vi "总磷总氮通讯.vi"() -> ()   [LabVIEW 2016, in "斯坦道总氮.lvlib"]
uses:
  <vilib>/Utility/config.llb/NI_LVConfig.lvlib
  <vilib>/Plasmionique/MB Master/MB_Master/MB_Master.lvclass
  <vilib>/Plasmionique/MB Master/MB Master.lvlib
  <vilib>/NI/Modbus Library/API/Wrapper/API Main.lvlib
  <vilib>/NI/Modbus Library/API/Slave/Modbus Slave.lvclass
  <vilib>/NI/Modbus Library/API/Wrapper/Create TCP Slave.vi
  <vilib>/ptbypt/NI_PtbyPt.lvlib
  <vilib>/Utility/config.llb/Write Key (Boolean).vi
  <vilib>/Utility/config.llb/Write Key (String).vi
panel:
  out "氨氮状态告警区":u16[](array[numeric])
  out "氨氮测量数据区":u16[](array[numeric])
  out "COD测量数据区":u16[](array[numeric])
  out "COD状态告警区":u16[](array[numeric])
  out "总氮测量数据区":u16[](array[numeric])
  out "总氮状态告警区":u16[](array[numeric])
  out "总磷状态告警区":u16[](array[numeric])
  out "总磷测量数据区":u16[](array[numeric])
  out "状态告警区":T1 {"告警代码" items=["无告警", "缺试剂告警", "缺水样告警", "缺蒸馏水告警", "缺标液告警", "仪表漏液告警", "标定异常告警", "超量程告警", "加热异常", "低试剂预警", "超上限告警", "超下限告警", "仪表内部其他异常", "滴定异常告警", "电极异常告警", "量程切换告警", "参数设置告警", "PH电极电位异常", "电导率电极异常", "浊度光度异常", "溶解氧电极异常", "溶解氧光强异常", "温度异常告警", "PH异常告警", "溶解氧异常告警", "电导率异常告警", "浊度异常告警", "叶绿素异常告警", "藻密度异常告警", "蓝绿藻异常告警", "ORP异常告警", "氨氮异常告警", "清洁刷异常告警", "SD卡异常告警", "蓝牙异常告警", "Wifi异常告警", "流程异常告警"]; "故障代码" items=["无故障", "电机故障", "温度故障", "通讯故障", "滴定故障"]}
  out "测量数据区":T2 {"单位" items=["ug/L", "mg/L", "ppm", "mg/m3", "cm", "ppb", "ug/m3", "%", "nmol/mol", "umol/mol", "MPN/L", "MPN/100ml", "ng/m3", "NTU", "无量纲", "ms/cm", "us/cm", "℃", "mV", "万个/L"]}
  out "status":bool
  out "关键参数区":T3
  in  "读关键参数区":bool
  in  "读状态告警区":bool
  in  "读测量数据区":bool
  in  "站号":u16(ring) items=["总磷"=1, "氨氮"=3]
  in  "停止":bool
  in  "启动":bool
  in  "控制命令":u16(ring) items=["启动测量"=1, "标样核查"=2, "零点核查"=3, "跨度核查"=4, "空白测试"=5, "平行样测试"=6, "加标回收"=7, "空白校准"=8, "标样校准"=9, "初始化（清洗）"=10, "停止测试"=11, "仪器重启"=12, "校时"=13, "模式设置"=14, "测量间隔设置"=15]
  in  "控制命令参数":u16[](array[numeric]) format="%04xH"
  in  "VISA Resource":refnum<visa-resource-name>
  in  "启用模块":bool
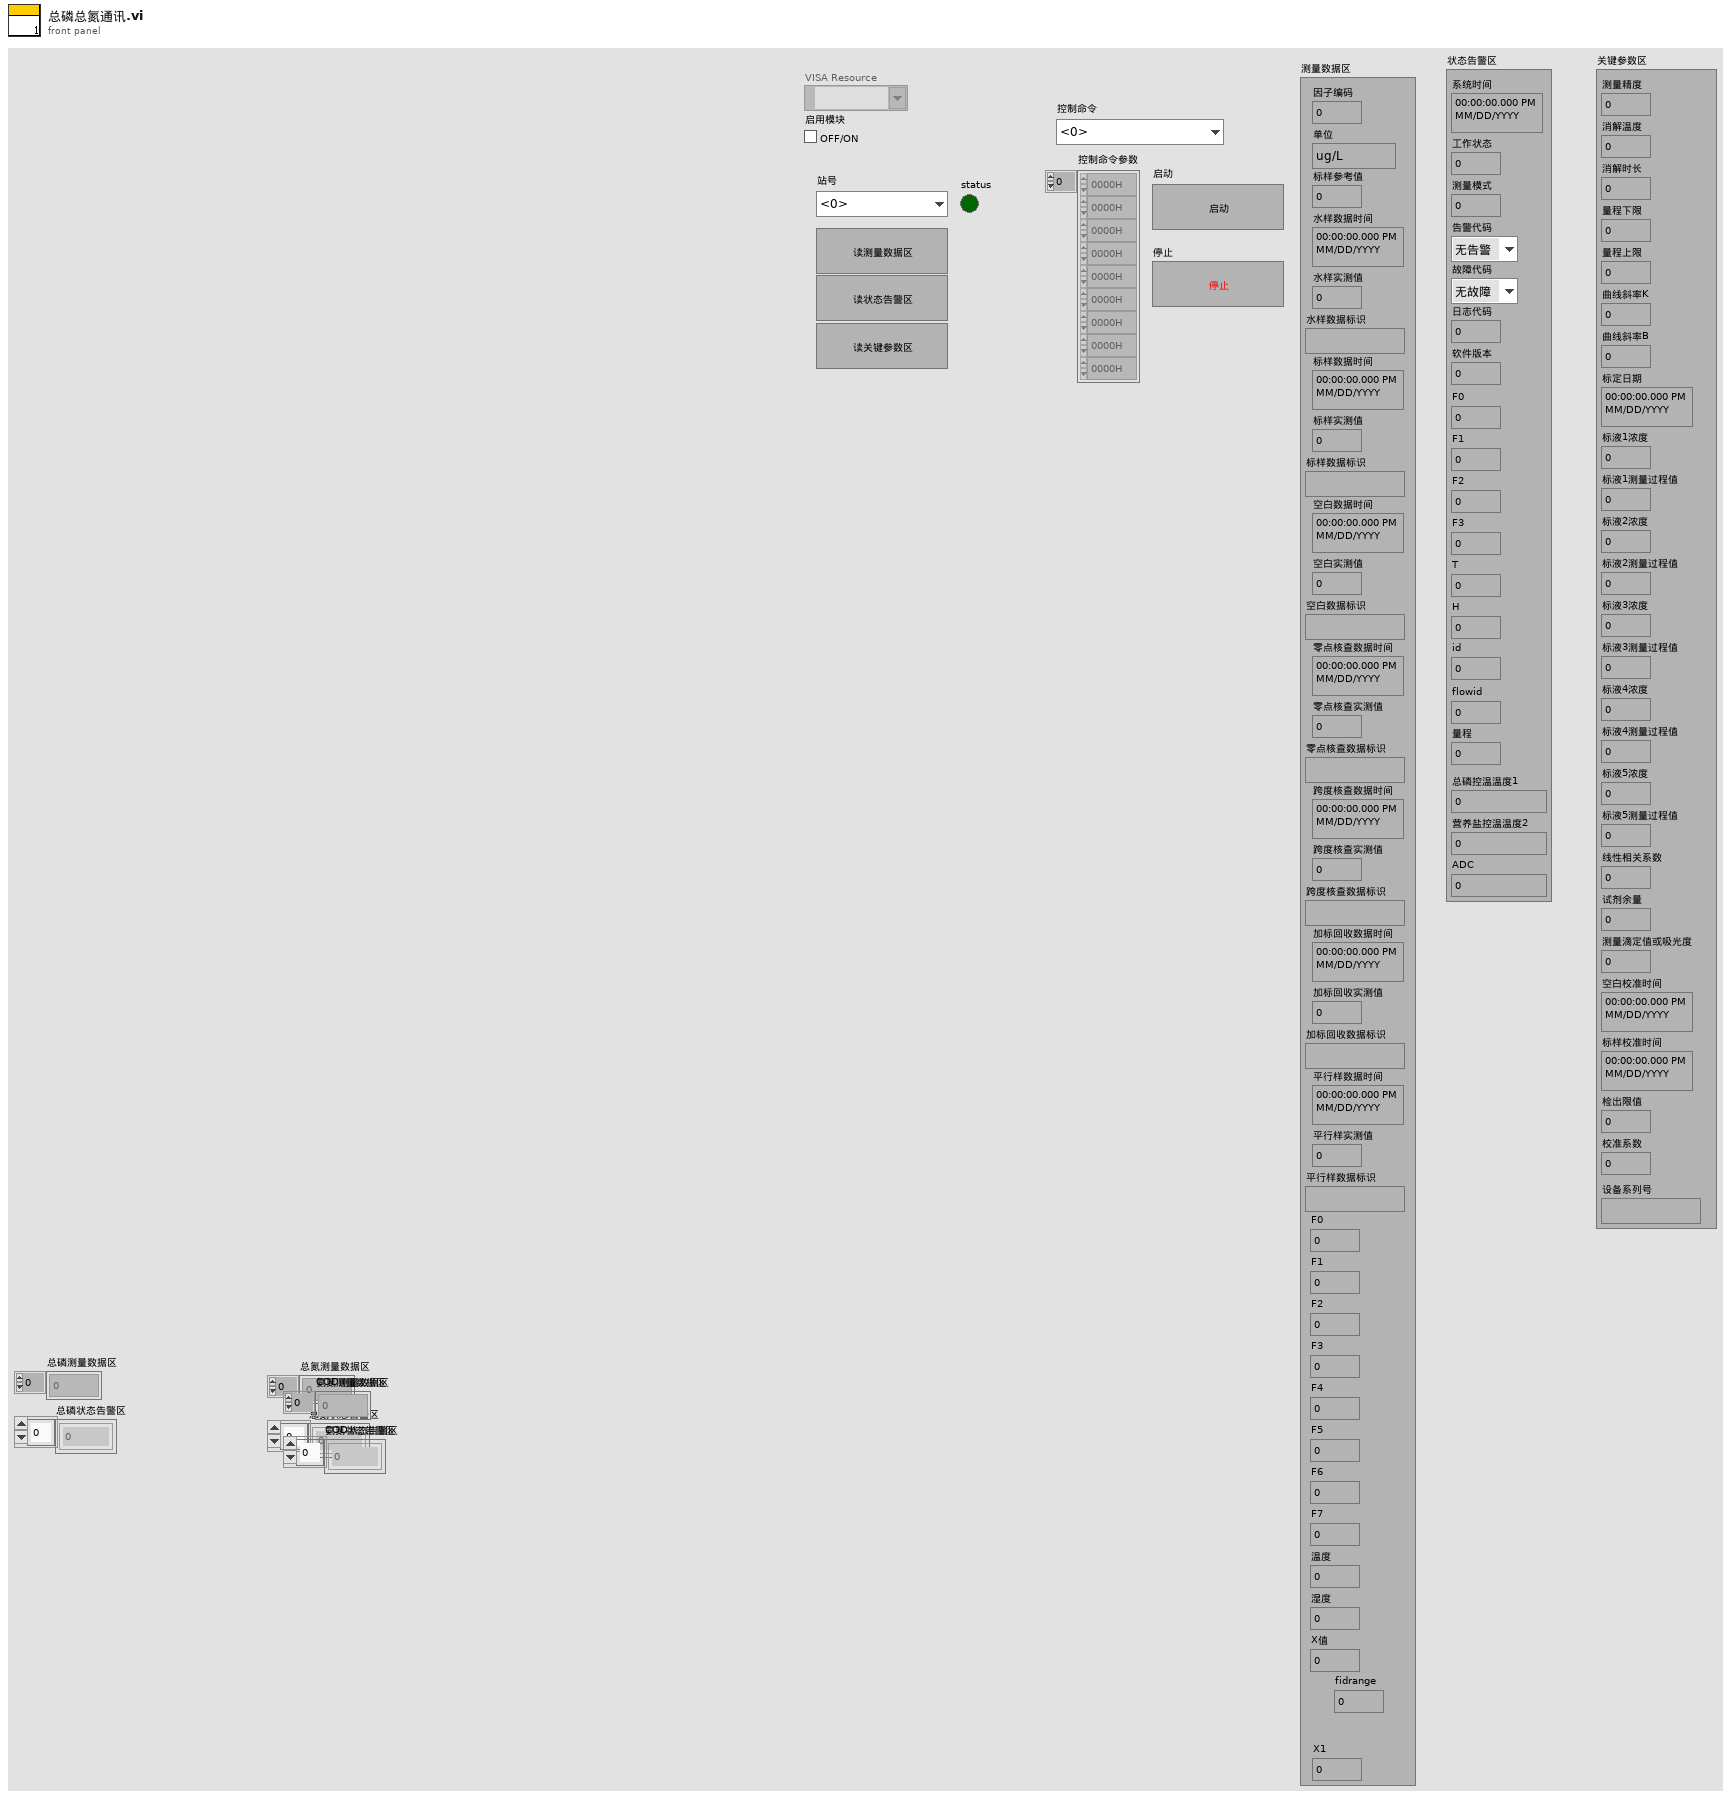
[diagram p1: front panel]
types:
  T1 = cluster{"系统时间":timestamp, "工作状态":u16, "测量模式":u16, "告警代码":u16, "故障代码":u16, "日志代码":u16, "软件版本":u16, "F0":sgl, "F1":sgl, "F2":sgl, "F3":sgl, "T":sgl, "H":sgl, "id":u16, "flowid":u16, "量程":u16, "总磷控温温度1":sgl, "营养盐控温温度2":sgl, "ADC":sgl}
  T2 = cluster{"因子编码":u32, "单位":u16, "标样参考值":sgl, "水样数据时间":timestamp, "水样实测值":sgl, "水样数据标识":string, "标样数据时间":timestamp, "标样实测值":sgl, "标样数据标识":string, "空白数据时间":timestamp, "空白实测值":sgl, "空白数据标识":string, "零点核查数据时间":timestamp, "零点核查实测值":sgl, "零点核查数据标识":string, "跨度核查数据时间":timestamp, "跨度核查实测值":sgl, "跨度核查数据标识":string, "加标回收数据时间":timestamp, "加标回收实测值":sgl, "加标回收数据标识":string, "平行样数据时间":timestamp, "平行样实测值":sgl, "平行样数据标识":string, "F0":sgl, "F1":sgl, "F2":sgl, "F3":sgl, "F4":sgl, "F5":sgl, "F6":sgl, "F7":sgl, "温度":sgl, "湿度":sgl, "X值":sgl, "fidrange":u16, "X1":sgl}
  T3 = cluster{"测量精度":u16, "消解温度":u16, "消解时长":u16, "量程下限":sgl, "量程上限":sgl, "曲线斜率K":sgl, "曲线斜率B":sgl, "标定日期":timestamp, "标液1浓度":sgl, "标液1测量过程值":sgl, "标液2浓度":sgl, "标液2测量过程值":sgl, "标液3浓度":sgl, "标液3测量过程值":sgl, "标液4浓度":sgl, "标液4测量过程值":sgl, "标液5浓度":sgl, "标液5测量过程值":sgl, "线性相关系数":sgl, "试剂余量":u32, "测量滴定值或吸光度":sgl, "空白校准时间":timestamp, "标样校准时间":timestamp, "检出限值":sgl, "校准系数":sgl, "设备系列号":string}
  T4 = cluster{"系统时间":timestamp, "工作状态":u16, "测量模式":enum16{"待机", "连续模式", "周期模式", "定点模式", "受控模式", "手动模式"}, "告警代码":u16, "故障代码":u16, "日志代码":u16, "软件版本":u16, "F0":sgl, "F1":sgl, "F2":sgl, "F3":sgl, "T":sgl, "H":sgl, "id":u16, "flowid":u16, "量程":u16, "总磷控温温度1":sgl, "营养盐控温温度2":sgl, "ADC":sgl}
  T5 = cluster{"因子编码":u32, "单位":u16, "标样参考值":sgl, "水样数据时间":timestamp, "水样实测值":sgl, "水样数据标识":string, "标样数据时间":timestamp, "标样实测值":sgl, "标样数据标识":string, "空白数据时间":timestamp, "空白实测值":sgl, "空白数据标识":string, "零点核查数据时间":timestamp, "零点核查实测值":sgl, "零点核查数据标识":string, "跨度核查数据时间":timestamp, "跨度核查实测值":sgl, "跨度核查数据标识":string, "加标回收数据时间":timestamp, "加标回收实测值":sgl, "加标回收数据标识":string, "平行样数据时间":timestamp, "平行样实测值":sgl, "平行样数据标识":string, "F0":sgl, "F1":sgl, "F2":sgl, "F3":sgl, "F4":sgl, "F5":sgl, "F6":sgl, "F7":sgl, "温度":sgl, "湿度":sgl, "X值":sgl, "fidrange":u16, "X1值":sgl}
  T6 = cluster{"因子编码":u32, "单位":u16, "标样参考值":sgl, "水样数据时间":timestamp, "水样实测值":sgl, "水样数据标识":string, "标样数据时间":timestamp, "标样实测值":sgl, "标样数据标识":string, "空白数据时间":timestamp, "空白实测值":sgl, "空白数据标识":string, "零点核查数据时间":timestamp, "零点核查实测值":sgl, "零点核查数据标识":string, "跨度核查数据时间":timestamp, "跨度核查实测值":sgl, "跨度核查数据标识":string, "加标回收数据时间":timestamp, "加标回收实测值":sgl, "加标回收数据标识":string, "平行样数据时间":timestamp, "平行样实测值":sgl, "平行样数据标识":string, "F0":sgl, "F1":sgl, "F2":sgl, "F3":sgl, "F4":sgl, "F5":sgl, "F6":sgl, "F7":sgl, "温度":sgl, "湿度":sgl, "X值":sgl, "fidrange":u16, "X1值":sgl}[]
  T7 = cluster{"测量精度":u16, "消解温度":u16, "消解时长":u16, "量程下限":sgl, "量程上限":sgl, "曲线斜率K":sgl, "曲线斜率B":sgl, "标定日期":timestamp, "标液1浓度":sgl, "标液1测量过程值":sgl, "标液2浓度":sgl, "标液2测量过程值":sgl, "标液3浓度":sgl, "标液3测量过程值":sgl, "标液4浓度":sgl, "标液4测量过程值":sgl, "标液5浓度":sgl, "标液5测量过程值":sgl, "线性相关系数":sgl, "试剂余量":u32, "测量滴定值或吸光度":sgl, "空白校准时间":timestamp, "标样校准时间":timestamp, "检出限值":sgl, "校准系数":sgl, "设备系列号":string}[]
  T8 = cluster{"系统时间":timestamp, "工作状态":u16, "测量模式":enum16{"待机", "连续模式", "周期模式", "定点模式", "受控模式", "手动模式"}, "告警代码":u16, "故障代码":u16, "日志代码":u16, "软件版本":u16, "F0":sgl, "F1":sgl, "F2":sgl, "F3":sgl, "T":sgl, "H":sgl, "id":u16, "flowid":u16, "量程":u16, "总磷控温温度1":sgl, "营养盐控温温度2":sgl, "ADC":sgl}[]
  T9 = typedef "总磷交互.ctl" = cluster{"状态告警区":cluster{"系统时间":timestamp, "工作状态":u16, "测量模式":enum16{"待机", "连续模式", "周期模式", "定点模式", "受控模式", "手动模式"}, "告警代码":u16, "故障代码":u16, "日志代码":u16, "软件版本":u16, "F0":sgl, "F1":sgl, "F2":sgl, "F3":sgl, "T":sgl, "H":sgl, "id":u16, "flowid":u16, "量程":u16, "总磷控温温度1":sgl, "营养盐控温温度2":sgl, "ADC":sgl}, "平台试剂余量百分比":sgl, "总磷关键参数":T10}
  T10 = typedef "关键参数.ctl" = cluster{"测量量程":sgl, "测量检出限":sgl, "测量精度":sgl, "测量间隔":sgl, "消解温度":sgl, "消解时长":sgl, "三项式系数":sgl, "二次多项式系数":sgl, "曲线斜率":sgl, "曲线截距":sgl, "线性相关系数":sgl, "空白校准时间":timestamp, "标样校准时间":timestamp, "测量信号值":sgl, "稀释倍数":sgl, "空白标定系数":sgl, "量程系数":sgl}
  T11 = typedef "斯坦道总氮.lvlib/关键参数.ctl" = cluster{"测量量程":sgl, "测量检出限":sgl, "测量精度":sgl, "测量间隔":sgl, "消解温度":sgl, "消解时长":sgl, "三项式系数":sgl, "二次多项式系数":sgl, "曲线斜率":sgl, "曲线截距":sgl, "线性相关系数":sgl, "空白校准时间":timestamp, "标样校准时间":timestamp, "测量信号值":sgl, "稀释倍数":sgl, "空白标定系数":sgl, "量程系数":sgl}
  T12 = typedef "总氮交互.ctl" = cluster{"状态告警区":cluster{"系统时间":timestamp, "工作状态":u16, "测量模式":enum16{"待机", "连续模式", "周期模式", "定点模式", "受控模式", "手动模式"}, "告警代码":u16, "故障代码":u16, "日志代码":u16, "软件版本":u16, "F0":sgl, "F1":sgl, "F2":sgl, "F3":sgl, "T":sgl, "H":sgl, "id":u16, "flowid":u16, "量程":u16, "总磷控温温度1":sgl, "营养盐控温温度2":sgl, "ADC":sgl}, "平台试剂余量百分比":sgl, "总氮关键参数":T10}
  T13 = typedef "氨氮交互.ctl" = cluster{"状态告警区":cluster{"系统时间":timestamp, "工作状态":u16, "测量模式":enum16{"待机", "连续模式", "周期模式", "定点模式", "受控模式", "手动模式"}, "告警代码":u16, "故障代码":u16, "日志代码":u16, "软件版本":u16, "F0":sgl, "F1":sgl, "F2":sgl, "F3":sgl, "T":sgl, "H":sgl, "id":u16, "flowid":u16, "量程":u16, "总磷控温温度1":sgl, "营养盐控温温度2":sgl, "ADC":sgl}, "平台试剂余量百分比":sgl, "氨氮关键参数":T10}
  T14 = typedef "CODCr交互.ctl" = cluster{"状态告警区":cluster{"系统时间":timestamp, "工作状态":u16, "测量模式":enum16{"待机", "连续模式", "周期模式", "定点模式", "受控模式", "手动模式"}, "告警代码":u16, "故障代码":u16, "日志代码":u16, "软件版本":u16, "F0":sgl, "F1":sgl, "F2":sgl, "F3":sgl, "T":sgl, "H":sgl, "id":u16, "flowid":u16, "量程":u16, "总磷控温温度1":sgl, "营养盐控温温度2":sgl, "ADC":sgl}, "平台试剂余量百分比":sgl, "CODcr关键参数":T10}
  T15 = typedef "NI_LVConfig.lvlib/Config Data RefNum.ctl" = refnum<k1>
  T16 = enum8{"Enabled", "Disabled", "Disabled and Grayed Out"}
  T17 = cluster{"时间标识":timestamp, "设备":string, "日志信息":string, "备注":string}
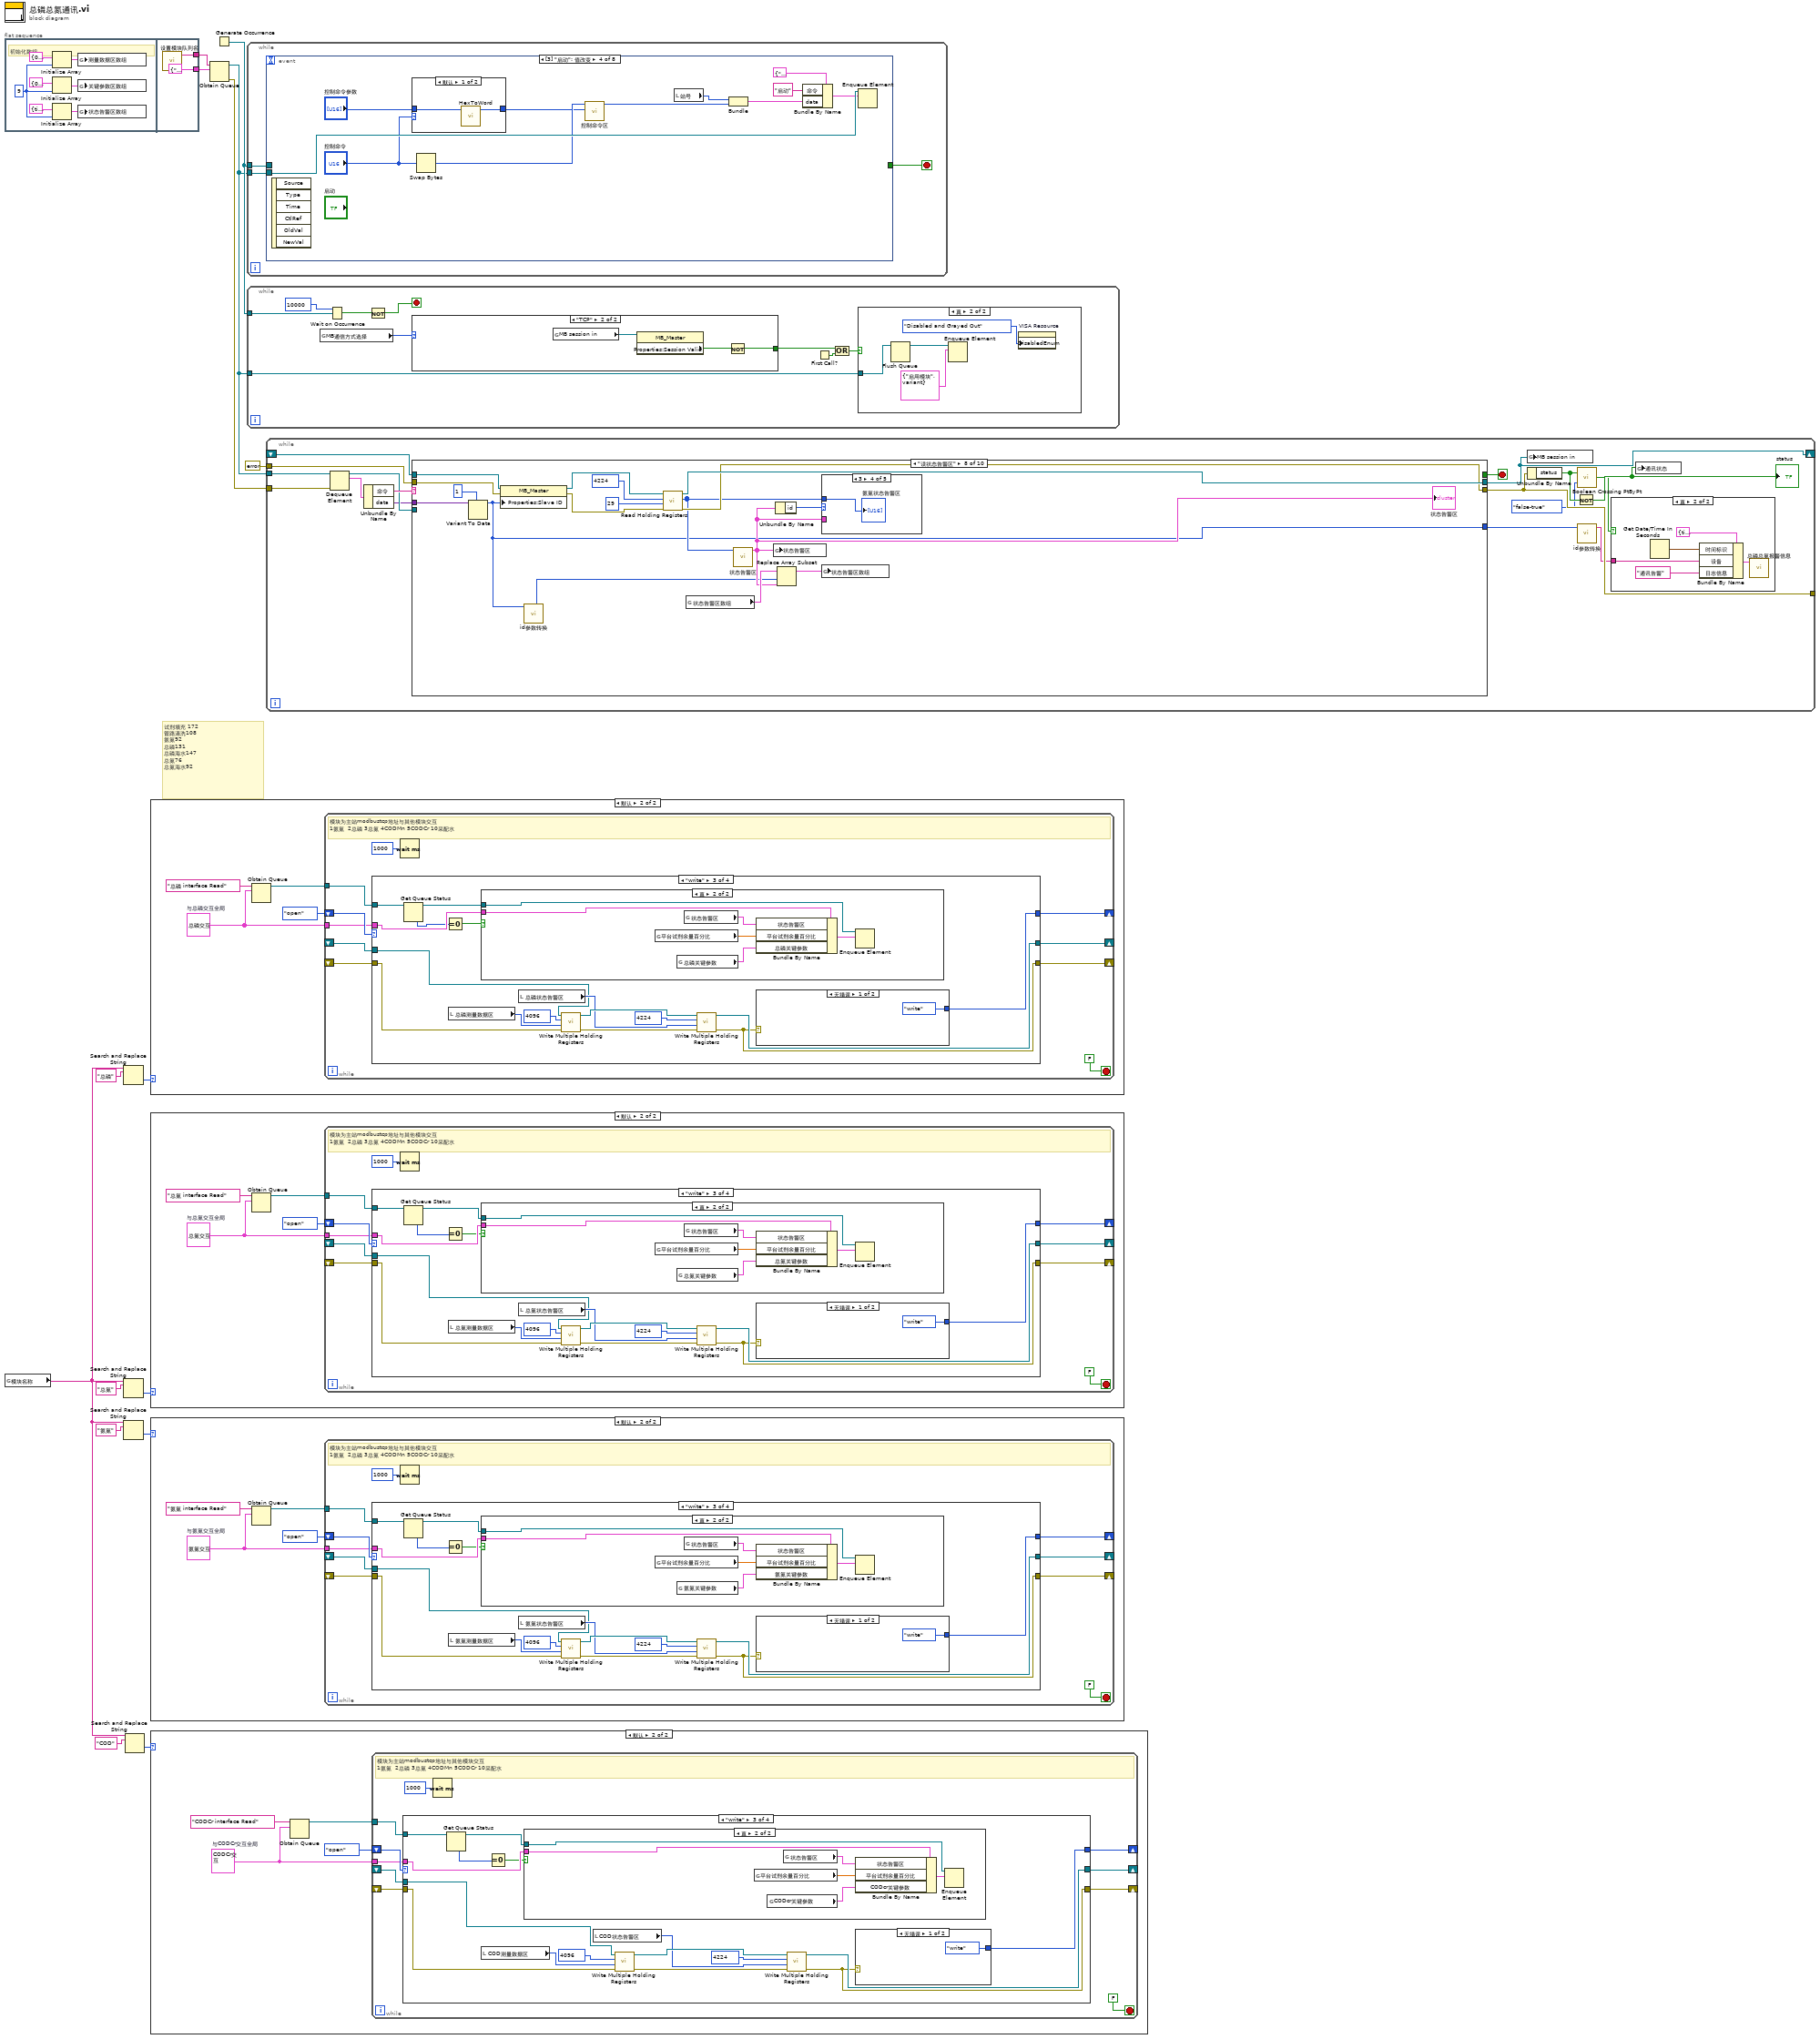
[diagram p0: block diagram]
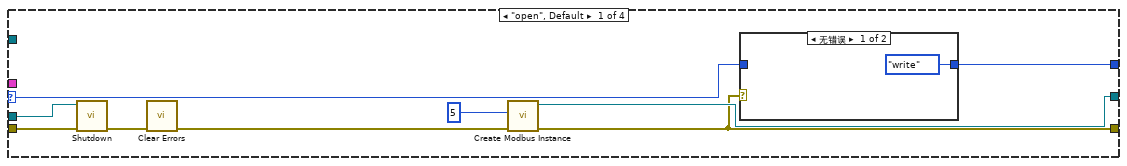
[diagram p3: hidden frame]
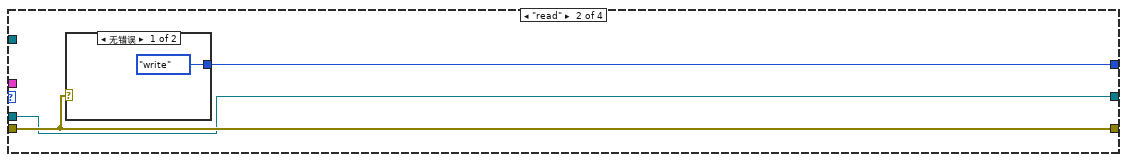
[diagram p5: hidden frame]
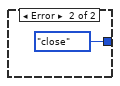
[diagram p6: hidden frame]
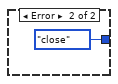
[diagram p8: hidden frame]
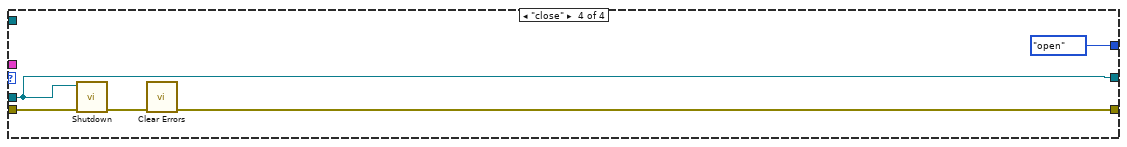
[diagram p9: hidden frame]
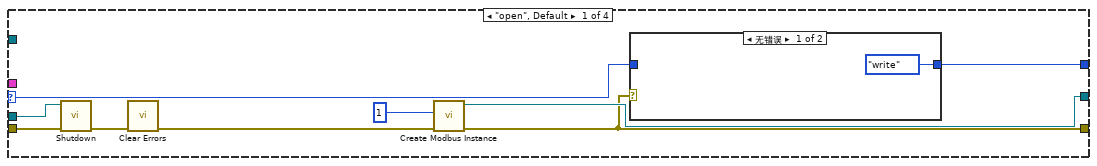
[diagram p11: hidden frame]
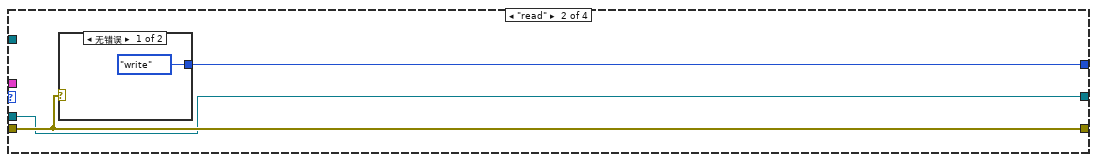
[diagram p13: hidden frame]
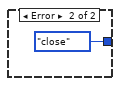
[diagram p14: hidden frame]
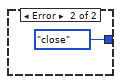
[diagram p16: hidden frame]
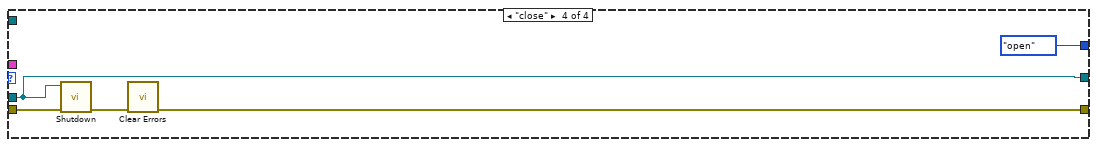
[diagram p17: hidden frame]
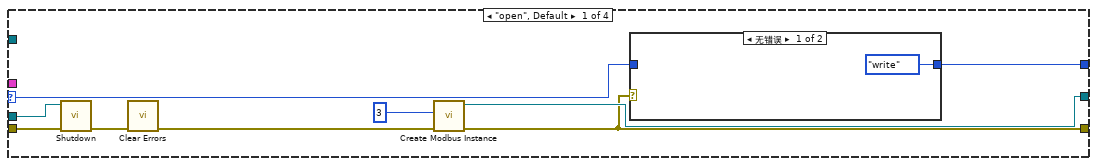
[diagram p19: hidden frame]
diagram:
  # "试剂填充 172 \n管路清洗108\n氨氮92\n总磷131\n总磷海水147\n总氮76\n总氮海水92"
  n1 = flat-sequence {
    tunnel: [cluster{"命令":string, "data":variant} {"命令"="", "data"=variant}] -> w15
    tunnel: [w23] -> w10
    frame #0 {
      w16 = 9 ("维数大小")
      # "初始化数组"
      n2 = Initialize Array(T5 {"因子编码"=0, "单位"=0, "标样参考值"=0.0, "水样数据时间"=timestamp(0 s since 1904-01-01), "水样实测值"=0.0, "水样数据标识"="", "标样数据时间"=timestamp(0 s since 1904-01-01), "标样实测值"=0.0, "标样数据标识"="", "空白数据时间"=timestamp(0 s since 1904-01-01), "空白实测值"=0.0, "空白数据标识"="", "零点核查数据时间"=timestamp(0 s since 1904-01-01), "零点核查实测值"=0.0, "零点核查数据标识"="", "跨度核查数据时间"=timestamp(0 s since 1904-01-01), "跨度核查实测值"=0.0, "跨度核查数据标识"="", "加标回收数据时间"=timestamp(0 s since 1904-01-01), "加标回收实测值"=0.0, "加标回收数据标识"="", "平行样数据时间"=timestamp(0 s since 1904-01-01), "平行样实测值"=0.0, "平行样数据标识"="", "F0"=0.0, "F1"=0.0, "F2"=0.0, "F3"=0.0, "F4"=0.0, "F5"=0.0, "F6"=0.0, "F7"=0.0, "温度"=0.0, "湿度"=0.0, "X值"=0.0, "fidrange"=0, "X1值"=0.0} ("测量数据区"), w16) -> (w22:T6)
      n3 = Initialize Array(T3 {"测量精度"=0, "消解温度"=0, "消解时长"=0, "量程下限"=0.0, "量程上限"=0.0, "曲线斜率K"=0.0, "曲线斜率B"=0.0, "标定日期"=timestamp(0 s since 1904-01-01), "标液1浓度"=0.0, "标液1测量过程值"=0.0, "标液2浓度"=0.0, "标液2测量过程值"=0.0, "标液3浓度"=0.0, "标液3测量过程值"=0.0, "标液4浓度"=0.0, "标液4测量过程值"=0.0, "标液5浓度"=0.0, "标液5测量过程值"=0.0, "线性相关系数"=0.0, "试剂余量"=0, "测量滴定值或吸光度"=0.0, "空白校准时间"=timestamp(0 s since 1904-01-01), "标样校准时间"=timestamp(0 s since 1904-01-01), "检出限值"=0.0, "校准系数"=0.0, "设备系列号"=""} ("关键参数区"), w16) -> (w20:T7)
      n4 = Initialize Array(T4 {"系统时间"=timestamp(0 s since 1904-01-01), "工作状态"=0, "测量模式"=enum."待机", "告警代码"=0, "故障代码"=0, "日志代码"=0, "软件版本"=0, "F0"=0.0, "F1"=0.0, "F2"=0.0, "F3"=0.0, "T"=0.0, "H"=0.0, "id"=0, "flowid"=0, "量程"=0, "总磷控温温度1"=0.0, "营养盐控温温度2"=0.0, "ADC"=0.0} ("状态告警区"), w16) -> (w19:T8)
      n5 = global write "VAR总磷总氮全局变量.vi" "测量数据区数组"(w22) -> ()
      n6 = global write "VAR总磷总氮全局变量.vi" "关键参数区数组"(w20) -> ()
      n7 = global write "VAR总磷总氮全局变量.vi" "状态告警区数组"(w19) -> ()
    }
    frame #1 {
      n8 = call "设置模块队列名.vi"() -> ("Msg"=w23:string)  [unwired: 5 in]
    }
  }
  n9 = global read "VAR总磷总氮全局变量.vi" "模块名称"() -> (w3:string)
  n10 = Search and Replace String(input string=w3, search string="总磷" ("搜索字符串")) -> (offset past replacement=w8:i32)  [unwired: 6 in, 3 out]
  n11 = Search and Replace String(input string=w3, search string="总氮" ("搜索字符串")) -> (offset past replacement=w6:i32)  [unwired: 6 in, 3 out]
  n12 = Search and Replace String(input string=w3, search string="氨氮" ("搜索字符串")) -> (offset past replacement=w4:i32)  [unwired: 6 in, 3 out]
  n13 = Search and Replace String(input string=w3, search string="COD" ("搜索字符串")) -> (offset past replacement=w1:i32)  [unwired: 6 in, 3 out]
  n14 = case shown="默认" w8 {
    frame -1 {
    }
    frame Default {
      w25 = T9 {"状态告警区"={"系统时间"=timestamp(0 s since 1904-01-01), "工作状态"=0, "测量模式"=enum."待机", "告警代码"=0, "故障代码"=0, "日志代码"=0, "软件版本"=0, "F0"=0.0, "F1"=0.0, "F2"=0.0, "F3"=0.0, "T"=0.0, "H"=0.0, "id"=0, "flowid"=0, "量程"=0, "总磷控温温度1"=0.0, "营养盐控温温度2"=0.0, "ADC"=0.0}, "平台试剂余量百分比"=0.0, "总磷关键参数"={"测量量程"=0.0, "测量检出限"=0.0, "测量精度"=0.0, "测量间隔"=0.0, "消解温度"=0.0, "消解时长"=0.0, "三项式系数"=0.0, "二次多项式系数"=0.0, "曲线斜率"=0.0, "曲线截距"=0.0, "线性相关系数"=0.0, "空白校准时间"=timestamp(0 s since 1904-01-01), "标样校准时间"=timestamp(0 s since 1904-01-01), "测量信号值"=0.0, "稀释倍数"=0.0, "空白标定系数"=0.0, "量程系数"=0.0}}  # 与总磷交互全局
      n15 = Obtain Queue(name (unnamed)="总磷 interface Read" ("写入方名称"), element data type=w25) -> (queue out=w26:refnum<queue>)  [unwired: 3 in, 2 out]
      n16 = while {
        shift-right: [w36] -> _
        shift-left: _ -> [w38]
        shift-right: [w35] -> _
        shift-left: _ -> [w37]
        shift-right: [w32] -> _
        shift-left: enum16{"open", "read", "write", "close"}."open" -> [w33]
        tunnel: w26 -> [w30]
        tunnel: w25 -> [w29]
        stop <- FALSE stop-if-true
        # "模块为主站modbustcp地址与其他模块交互\n1氨氮  2总磷 3总氮 4CODMn 5CODCr 10采配水"
        n17 = case shown="\"write\"" w33 {
          selector: w33 -> [w47 _ _ _]
          tunnel: w38 -> [w41 w50 w61 w81]
          tunnel: w37 -> [w40 w51 w60 w80]
          tunnel: [w44 w50 w66 w81] -> w36
          tunnel: [w43 w51 w65 w83] -> w35
          tunnel: [w46 w52 w70 enum16{"open", "read", "write", "close"}."open"] -> w32
          tunnel: w30 -> [_ _ w59 _]
          tunnel: w29 -> [_ _ w58 _]
          frame "open", Default {
            n18 = call-dynamic "Shutdown.vi"("error in"=w40, "Modbus slave in"=w41) -> ("error out"=w39:errorcluster)  [unwired: 9 in]
            n19 = call <vilib>:"Clear Errors.vi"("error in (no error)"=w39) -> ("error out"=w42:errorcluster)  [unwired: 5 in, 1 out]
            n20 = call-poly <vilib>:"Create Modbus Instance.vi"("error in"=w42, "port (502)"=u16 2) -> ("error out"=w43:errorcluster, "TCP slave instance"=w44:refnum<class "Modbus Slave.lvclass">)  [unwired: 8 in]
            n21 = case shown="无错误" w43 {
              tunnel: w47 -> [_ w49]
              tunnel: [enum16{"open", "read", "write", "close"}."write" w49] -> w46
              frame No Error {
              }
              frame Error {
              }
            }
          }
          frame "read" {
            n22 = case shown="无错误" w51 {
              tunnel: [enum16{"open", "read", "write", "close"}."write" enum16{"open", "read", "write", "close"}."close"] -> w52
              frame No Error {
              }
              frame Error {
              }
            }
          }
          frame "write" {
            n23 = Get Queue Status(queue=w59) -> (queue out=w57:refnum<queue>, # elements in queue=w56:i32)  [unwired: 2 in, 6 out]
            n24 = Equal To 0?(x=w56) -> (x = 0?=w55:bool)
            n25 = local read "总磷测量数据区"() -> (w64:u16[])
            n26 = case shown="真" w55 {
              tunnel: w58 -> [_ w73]
              tunnel: w57 -> [_ w71]
              frame False {
              }
              frame True {
                n27 = global read "VAR总磷总氮全局变量.vi" "平台试剂余量百分比"() -> (w75:sgl)
                n28 = global read "VAR总磷总氮全局变量.vi" "总磷关键参数"() -> (w76:T11)
                n29 = global read "VAR总磷总氮全局变量.vi" "状态告警区"() -> (w74:T4)
                n30 = Bundle By Name(cluster=w73, "状态告警区"=w74, "平台试剂余量百分比"=w75, "总磷关键参数"=w76) -> (w72:T9)
                n31 = Enqueue Element(queue=w71, element=w72) -> ()  [unwired: 2 in, 3 out]
              }
            }
            n32 = local read "总磷状态告警区"() -> (w62:u16[])
            n33 = call-dynamic "Write Multiple Holding Registers.vi"("error in"=w60, "registers to write"=w64, "starting address"=u16 4096, "Modbus slave in"=w61) -> ("error out"=w67:errorcluster, "Modbus slave out"=w68:refnum<class "Modbus Slave.lvclass">)  [unwired: 6 in]
            n34 = call-dynamic "Write Multiple Holding Registers.vi"("error in"=w67, "registers to write"=w62, "starting address"=u16 4224, "Modbus slave in"=w68) -> ("error out"=w65:errorcluster, "Modbus slave out"=w66:refnum<class "Modbus Slave.lvclass">)  [unwired: 6 in]
            n35 = case shown="无错误" w65 {
              tunnel: [enum16{"open", "read", "write", "close"}."write" enum16{"open", "read", "write", "close"}."close"] -> w70
              frame No Error {
              }
              frame Error {
              }
            }
          }
          frame "close" {
            n36 = call-dynamic "Shutdown.vi"("error in"=w80, "Modbus slave in"=w81) -> ("error out"=w79:errorcluster)  [unwired: 9 in]
            n37 = call <vilib>:"Clear Errors.vi"("error in (no error)"=w79) -> ("error out"=w83:errorcluster)  [unwired: 5 in, 1 out]
          }
        }
        n38 = Wait (ms)(milliseconds to wait=u32 1000 ("等待时间（毫秒）")) -> ()  [unwired: 1 out]
      }
    }
  }
  n39 = case shown="默认" w6 {
    frame -1 {
    }
    frame Default {
      w84 = T12 {"状态告警区"={"系统时间"=timestamp(0 s since 1904-01-01), "工作状态"=0, "测量模式"=enum."待机", "告警代码"=0, "故障代码"=0, "日志代码"=0, "软件版本"=0, "F0"=0.0, "F1"=0.0, "F2"=0.0, "F3"=0.0, "T"=0.0, "H"=0.0, "id"=0, "flowid"=0, "量程"=0, "总磷控温温度1"=0.0, "营养盐控温温度2"=0.0, "ADC"=0.0}, "平台试剂余量百分比"=0.0, "总氮关键参数"={"测量量程"=0.0, "测量检出限"=0.0, "测量精度"=0.0, "测量间隔"=0.0, "消解温度"=0.0, "消解时长"=0.0, "三项式系数"=0.0, "二次多项式系数"=0.0, "曲线斜率"=0.0, "曲线截距"=0.0, "线性相关系数"=0.0, "空白校准时间"=timestamp(0 s since 1904-01-01), "标样校准时间"=timestamp(0 s since 1904-01-01), "测量信号值"=0.0, "稀释倍数"=0.0, "空白标定系数"=0.0, "量程系数"=0.0}}  # 与总氮交互全局
      n40 = Obtain Queue(name (unnamed)="总氮 interface Read" ("写入方名称"), element data type=w84) -> (queue out=w85:refnum<queue>)  [unwired: 3 in, 2 out]
      n41 = while {
        shift-right: [w95] -> _
        shift-left: _ -> [w97]
        shift-right: [w94] -> _
        shift-left: _ -> [w96]
        shift-right: [w91] -> _
        shift-left: enum16{"open", "read", "write", "close"}."open" -> [w92]
        tunnel: w85 -> [w89]
        tunnel: w84 -> [w88]
        stop <- FALSE stop-if-true
        # "模块为主站modbustcp地址与其他模块交互\n1氨氮  2总磷 3总氮 4CODMn 5CODCr 10采配水"
        n42 = case shown="\"write\"" w92 {
          selector: w92 -> [w106 _ _ _]
          tunnel: w97 -> [w100 w109 w120 w140]
          tunnel: w96 -> [w99 w110 w119 w139]
          tunnel: [w103 w109 w125 w140] -> w95
          tunnel: [w102 w110 w124 w142] -> w94
          tunnel: [w105 w111 w129 enum16{"open", "read", "write", "close"}."open"] -> w91
          tunnel: w89 -> [_ _ w118 _]
          tunnel: w88 -> [_ _ w117 _]
          frame "open", Default {
            n43 = call-dynamic "Shutdown.vi"("error in"=w99, "Modbus slave in"=w100) -> ("error out"=w98:errorcluster)  [unwired: 9 in]
            n44 = call <vilib>:"Clear Errors.vi"("error in (no error)"=w98) -> ("error out"=w101:errorcluster)  [unwired: 5 in, 1 out]
            n45 = call-poly <vilib>:"Create Modbus Instance.vi"("error in"=w101, "port (502)"=u16 3) -> ("error out"=w102:errorcluster, "TCP slave instance"=w103:refnum<class "Modbus Slave.lvclass">)  [unwired: 8 in]
            n46 = case shown="无错误" w102 {
              tunnel: w106 -> [_ w108]
              tunnel: [enum16{"open", "read", "write", "close"}."write" w108] -> w105
              frame No Error {
              }
              frame Error {
              }
            }
          }
          frame "read" {
            n47 = case shown="无错误" w110 {
              tunnel: [enum16{"open", "read", "write", "close"}."write" enum16{"open", "read", "write", "close"}."close"] -> w111
              frame No Error {
              }
              frame Error {
              }
            }
          }
          frame "write" {
            n48 = Get Queue Status(queue=w118) -> (queue out=w116:refnum<queue>, # elements in queue=w115:i32)  [unwired: 2 in, 6 out]
            n49 = Equal To 0?(x=w115) -> (x = 0?=w114:bool)
            n50 = local read "总氮测量数据区"() -> (w123:u16[])
            n51 = case shown="真" w114 {
              tunnel: w116 -> [_ w131]
              tunnel: w117 -> [_ w130]
              frame False {
              }
              frame True {
                n52 = global read "VAR总磷总氮全局变量.vi" "平台试剂余量百分比"() -> (w134:sgl)
                n53 = global read "VAR总磷总氮全局变量.vi" "总氮关键参数"() -> (w135:T11)
                n54 = global read "VAR总磷总氮全局变量.vi" "状态告警区"() -> (w133:T4)
                n55 = Bundle By Name(cluster=w130, "状态告警区"=w133, "平台试剂余量百分比"=w134, "总氮关键参数"=w135) -> (w132:T12)
                n56 = Enqueue Element(queue=w131, element=w132) -> ()  [unwired: 2 in, 3 out]
              }
            }
            n57 = local read "总氮状态告警区"() -> (w121:u16[])
            n58 = call-dynamic "Write Multiple Holding Registers.vi"("error in"=w119, "registers to write"=w123, "starting address"=u16 4096, "Modbus slave in"=w120) -> ("error out"=w126:errorcluster, "Modbus slave out"=w127:refnum<class "Modbus Slave.lvclass">)  [unwired: 6 in]
            n59 = call-dynamic "Write Multiple Holding Registers.vi"("error in"=w126, "registers to write"=w121, "starting address"=u16 4224, "Modbus slave in"=w127) -> ("error out"=w124:errorcluster, "Modbus slave out"=w125:refnum<class "Modbus Slave.lvclass">)  [unwired: 6 in]
            n60 = case shown="无错误" w124 {
              tunnel: [enum16{"open", "read", "write", "close"}."write" enum16{"open", "read", "write", "close"}."close"] -> w129
              frame No Error {
              }
              frame Error {
              }
            }
          }
          frame "close" {
            n61 = call-dynamic "Shutdown.vi"("error in"=w139, "Modbus slave in"=w140) -> ("error out"=w138:errorcluster)  [unwired: 9 in]
            n62 = call <vilib>:"Clear Errors.vi"("error in (no error)"=w138) -> ("error out"=w142:errorcluster)  [unwired: 5 in, 1 out]
          }
        }
        n63 = Wait (ms)(milliseconds to wait=u32 1000 ("等待时间（毫秒）")) -> ()  [unwired: 1 out]
      }
    }
  }
  n64 = case shown="默认" w4 {
    frame -1 {
    }
    frame Default {
      w143 = T13 {"状态告警区"={"系统时间"=timestamp(0 s since 1904-01-01), "工作状态"=0, "测量模式"=enum."待机", "告警代码"=0, "故障代码"=0, "日志代码"=0, "软件版本"=0, "F0"=0.0, "F1"=0.0, "F2"=0.0, "F3"=0.0, "T"=0.0, "H"=0.0, "id"=0, "flowid"=0, "量程"=0, "总磷控温温度1"=0.0, "营养盐控温温度2"=0.0, "ADC"=0.0}, "平台试剂余量百分比"=0.0, "氨氮关键参数"={"测量量程"=0.0, "测量检出限"=0.0, "测量精度"=0.0, "测量间隔"=0.0, "消解温度"=0.0, "消解时长"=0.0, "三项式系数"=0.0, "二次多项式系数"=0.0, "曲线斜率"=0.0, "曲线截距"=0.0, "线性相关系数"=0.0, "空白校准时间"=timestamp(0 s since 1904-01-01), "标样校准时间"=timestamp(0 s since 1904-01-01), "测量信号值"=0.0, "稀释倍数"=0.0, "空白标定系数"=0.0, "量程系数"=0.0}}  # 与氨氮交互全局
      n65 = Obtain Queue(name (unnamed)="氨氮 interface Read" ("写入方名称"), element data type=w143) -> (queue out=w144:refnum<queue>)  [unwired: 3 in, 2 out]
      n66 = while {
        shift-right: [w154] -> _
        shift-left: _ -> [w156]
        shift-right: [w153] -> _
        shift-left: _ -> [w155]
        shift-right: [w150] -> _
        shift-left: enum16{"open", "read", "write", "close"}."open" -> [w151]
        tunnel: w144 -> [w148]
        tunnel: w143 -> [w147]
        stop <- FALSE stop-if-true
        # "模块为主站modbustcp地址与其他模块交互\n1氨氮  2总磷 3总氮 4CODMn 5CODCr 10采配水"
        n67 = case shown="\"write\"" w151 {
          selector: w151 -> [w165 _ _ _]
          tunnel: w156 -> [w159 w168 w179 w199]
          tunnel: w155 -> [w158 w169 w178 w198]
          tunnel: [w162 w168 w184 w199] -> w154
          tunnel: [w161 w169 w183 w201] -> w153
          tunnel: [w164 w170 w188 enum16{"open", "read", "write", "close"}."open"] -> w150
          tunnel: w148 -> [_ _ w175 _]
          tunnel: w147 -> [_ _ w177 _]
          frame "open", Default {
            n68 = call-dynamic "Shutdown.vi"("error in"=w158, "Modbus slave in"=w159) -> ("error out"=w157:errorcluster)  [unwired: 9 in]
            n69 = call <vilib>:"Clear Errors.vi"("error in (no error)"=w157) -> ("error out"=w160:errorcluster)  [unwired: 5 in, 1 out]
            n70 = call-poly <vilib>:"Create Modbus Instance.vi"("error in"=w160, "port (502)"=u16 1) -> ("error out"=w161:errorcluster, "TCP slave instance"=w162:refnum<class "Modbus Slave.lvclass">)  [unwired: 8 in]
            n71 = case shown="无错误" w161 {
              tunnel: w165 -> [_ w167]
              tunnel: [enum16{"open", "read", "write", "close"}."write" w167] -> w164
              frame No Error {
              }
              frame Error {
              }
            }
          }
          frame "read" {
            n72 = case shown="无错误" w169 {
              tunnel: [enum16{"open", "read", "write", "close"}."write" enum16{"open", "read", "write", "close"}."close"] -> w170
              frame No Error {
              }
              frame Error {
              }
            }
          }
          frame "write" {
            n73 = Get Queue Status(queue=w175) -> (queue out=w174:refnum<queue>, # elements in queue=w176:i32)  [unwired: 2 in, 6 out]
            n74 = Equal To 0?(x=w176) -> (x = 0?=w173:bool)
            n75 = local read "氨氮测量数据区"() -> (w182:u16[])
            n76 = case shown="真" w173 {
              tunnel: w174 -> [_ w190]
              tunnel: w177 -> [_ w189]
              frame False {
              }
              frame True {
                n77 = global read "VAR总磷总氮全局变量.vi" "平台试剂余量百分比"() -> (w193:sgl)
                n78 = global read "VAR总磷总氮全局变量.vi" "氨氮关键参数"() -> (w194:T11)
                n79 = global read "VAR总磷总氮全局变量.vi" "状态告警区"() -> (w192:T4)
                n80 = Bundle By Name(cluster=w189, "状态告警区"=w192, "平台试剂余量百分比"=w193, "氨氮关键参数"=w194) -> (w191:T13)
                n81 = Enqueue Element(queue=w190, element=w191) -> ()  [unwired: 2 in, 3 out]
              }
            }
            n82 = local read "氨氮状态告警区"() -> (w180:u16[])
            n83 = call-dynamic "Write Multiple Holding Registers.vi"("error in"=w178, "registers to write"=w182, "starting address"=u16 4096, "Modbus slave in"=w179) -> ("error out"=w185:errorcluster, "Modbus slave out"=w186:refnum<class "Modbus Slave.lvclass">)  [unwired: 6 in]
            n84 = call-dynamic "Write Multiple Holding Registers.vi"("error in"=w185, "registers to write"=w180, "starting address"=u16 4224, "Modbus slave in"=w186) -> ("error out"=w183:errorcluster, "Modbus slave out"=w184:refnum<class "Modbus Slave.lvclass">)  [unwired: 6 in]
            n85 = case shown="无错误" w183 {
              tunnel: [enum16{"open", "read", "write", "close"}."write" enum16{"open", "read", "write", "close"}."close"] -> w188
              frame No Error {
              }
              frame Error {
              }
            }
          }
          frame "close" {
            n86 = call-dynamic "Shutdown.vi"("error in"=w198, "Modbus slave in"=w199) -> ("error out"=w197:errorcluster)  [unwired: 9 in]
            n87 = call <vilib>:"Clear Errors.vi"("error in (no error)"=w197) -> ("error out"=w201:errorcluster)  [unwired: 5 in, 1 out]
          }
        }
        n88 = Wait (ms)(milliseconds to wait=u32 1000 ("等待时间（毫秒）")) -> ()  [unwired: 1 out]
      }
    }
  }
  n89 = case shown="默认" w1 {
    frame -1 {
    }
    frame Default {
      w203 = T14 {"状态告警区"={"系统时间"=timestamp(0 s since 1904-01-01), "工作状态"=0, "测量模式"=enum."待机", "告警代码"=0, "故障代码"=0, "日志代码"=0, "软件版本"=0, "F0"=0.0, "F1"=0.0, "F2"=0.0, "F3"=0.0, "T"=0.0, "H"=0.0, "id"=0, "flowid"=0, "量程"=0, "总磷控温温度1"=0.0, "营养盐控温温度2"=0.0, "ADC"=0.0}, "平台试剂余量百分比"=0.0, "CODcr关键参数"={"测量量程"=0.0, "测量检出限"=0.0, "测量精度"=0.0, "测量间隔"=0.0, "消解温度"=0.0, "消解时长"=0.0, "三项式系数"=0.0, "二次多项式系数"=0.0, "曲线斜率"=0.0, "曲线截距"=0.0, "线性相关系数"=0.0, "空白校准时间"=timestamp(0 s since 1904-01-01), "标样校准时间"=timestamp(0 s since 1904-01-01), "测量信号值"=0.0, "稀释倍数"=0.0, "空白标定系数"=0.0, "量程系数"=0.0}}  # 与CODCr交互全局
      n90 = Obtain Queue(name (unnamed)="CODCr interface Read" ("写入方名称"), element data type=w203) -> (queue out=w204:refnum<queue>)  [unwired: 3 in, 2 out]
      n91 = while {
        shift-right: [w213] -> _
        shift-left: _ -> [w215]
        shift-right: [w212] -> _
        shift-left: _ -> [w214]
        shift-right: [w209] -> _
        shift-left: enum16{"open", "read", "write", "close"}."open" -> [w210]
        tunnel: w204 -> [w207]
        tunnel: w203 -> [w206]
        stop <- FALSE stop-if-true
        # "模块为主站modbustcp地址与其他模块交互\n1氨氮  2总磷 3总氮 4CODMn 5CODCr 10采配水"
        n92 = case shown="\"write\"" w210 {
          selector: w210 -> [w224 _ _ _]
          tunnel: w215 -> [w218 w227 w238 w258]
          tunnel: w214 -> [w217 w228 w237 w257]
          tunnel: [w221 w227 w243 w258] -> w213
          tunnel: [w220 w228 w242 w260] -> w212
          tunnel: [w223 w229 w247 enum16{"open", "read", "write", "close"}."open"] -> w209
          tunnel: w207 -> [_ _ w234 _]
          tunnel: w206 -> [_ _ w236 _]
          frame "open", Default {
            n93 = call-dynamic "Shutdown.vi"("error in"=w217, "Modbus slave in"=w218) -> ("error out"=w216:errorcluster)  [unwired: 9 in]
            n94 = call <vilib>:"Clear Errors.vi"("error in (no error)"=w216) -> ("error out"=w219:errorcluster)  [unwired: 5 in, 1 out]
            n95 = call-poly <vilib>:"Create Modbus Instance.vi"("error in"=w219, "port (502)"=u16 5) -> ("error out"=w220:errorcluster, "TCP slave instance"=w221:refnum<class "Modbus Slave.lvclass">)  [unwired: 8 in]
            n96 = case shown="无错误" w220 {
              tunnel: w224 -> [_ w226]
              tunnel: [enum16{"open", "read", "write", "close"}."write" w226] -> w223
              frame No Error {
              }
              frame Error {
              }
            }
          }
          frame "read" {
            n97 = case shown="无错误" w228 {
              tunnel: [enum16{"open", "read", "write", "close"}."write" enum16{"open", "read", "write", "close"}."close"] -> w229
              frame No Error {
              }
              frame Error {
              }
            }
          }
          frame "write" {
            n98 = Get Queue Status(queue=w234) -> (queue out=w233:refnum<queue>, # elements in queue=w235:i32)  [unwired: 2 in, 6 out]
            n99 = local read "COD测量数据区"() -> (w241:u16[])
            n100 = Equal To 0?(x=w235) -> (x = 0?=w232:bool)
            n101 = case shown="真" w232 {
              tunnel: w233 -> [_ w249]
              tunnel: w236 -> [_ w248]
              frame False {
              }
              frame True {
                n102 = global read "VAR总磷总氮全局变量.vi" "平台试剂余量百分比"() -> (w252:sgl)
                n103 = global read "VAR总磷总氮全局变量.vi" "CODcr关键参数"() -> (w253:T11)
                n104 = global read "VAR总磷总氮全局变量.vi" "状态告警区"() -> (w251:T4)
                n105 = Bundle By Name(cluster=w248, "状态告警区"=w251, "平台试剂余量百分比"=w252, "CODcr关键参数"=w253) -> (w250:T14)
                n106 = Enqueue Element(queue=w249, element=w250) -> ()  [unwired: 2 in, 3 out]
              }
            }
            n107 = local read "COD状态告警区"() -> (w239:u16[])
            n108 = call-dynamic "Write Multiple Holding Registers.vi"("error in"=w237, "registers to write"=w241, "starting address"=u16 4096, "Modbus slave in"=w238) -> ("error out"=w244:errorcluster, "Modbus slave out"=w245:refnum<class "Modbus Slave.lvclass">)  [unwired: 6 in]
            n109 = call-dynamic "Write Multiple Holding Registers.vi"("error in"=w244, "registers to write"=w239, "starting address"=u16 4224, "Modbus slave in"=w245) -> ("error out"=w242:errorcluster, "Modbus slave out"=w243:refnum<class "Modbus Slave.lvclass">)  [unwired: 6 in]
            n110 = case shown="无错误" w242 {
              tunnel: [enum16{"open", "read", "write", "close"}."write" enum16{"open", "read", "write", "close"}."close"] -> w247
              frame No Error {
              }
              frame Error {
              }
            }
          }
          frame "close" {
            n111 = call-dynamic "Shutdown.vi"("error in"=w257, "Modbus slave in"=w258) -> ("error out"=w256:errorcluster)  [unwired: 9 in]
            n112 = call <vilib>:"Clear Errors.vi"("error in (no error)"=w256) -> ("error out"=w260:errorcluster)  [unwired: 5 in, 1 out]
          }
        }
        n113 = Wait (ms)(milliseconds to wait=u32 1000 ("等待时间（毫秒）")) -> ()  [unwired: 1 out]
      }
    }
  }
  n114 = Obtain Queue(name (unnamed)=w10, element data type=w15) -> (queue out=w11:refnum<queue>, error out=w14:errorcluster)  [unwired: 3 in, 1 out]
  n115 = Generate Occurrence() -> (w12:refnum<k4>)
  n116 = while {
    tunnel: w11 -> [w263]
    tunnel: w12 -> [w261]
    stop <- w262 stop-if-true
    n117 = event shown="[3] \"启动\": 值改变" {
      selector: _ -> [_ _ _ _ _ _ _ _]
      dyn-events: _ -> [_ _ _ _ _ _ _ _]
      timeout: _ -> [_ _ _ _ _ _ _ _]
      tunnel: w263 -> [_ _ _ w294 w301 w307 w312 w317]
      tunnel: [_ _ _ _ "停止" _ _ _] -> w262
      tunnel: w261 -> [_ _ _ _ w298 _ _ _]
      event Timeout {
        n118 = event-data() -> ()  [unwired: 1 in, 3 out]
      }
      event "启用模块": Value Change {
        n119 = event-data() -> ("NewVal"=w264:bool)  [unwired: 1 in, 5 out]
        n120 = call <vilib>:"Application Directory.vi"() -> ("Application Directory"=w266:path)
        n121 = Build Path(base path=w266, name or relative path="data\\set.ini" ("名称或相对路径")) -> (appended path=w267:path)
        n122 = call <vilib>:"Open Config Data.vi"("configuration file path"=w267) -> ("error out"=w273:errorcluster, "refnum"=w272:T15)  [unwired: 8 in, 1 out]
        n123 = call-poly <vilib>:"Write Key.vi"("section"="总磷总氮", "error in (no error)"=w273, "value"=w264, "key"="模块启用", "refnum"=w272) -> ("error out"=w269:errorcluster, "refnum out"=w265:T15)  [unwired: 4 in, 1 out]
        n124 = call <vilib>:"Close Config Data.vi"("error in (no error)"=w269, "refnum"=w265) -> ()  [unwired: 8 in, 2 out]
      }
      event "VISA Resource": Value Change {
        n125 = event-data() -> ()  [unwired: 1 in, 6 out]
        n126 = call <vilib>:"Application Directory.vi"() -> ("Application Directory"=w276:path)
        n127 = Build Path(base path=w276, name or relative path="data\\set.ini" ("名称或相对路径")) -> (appended path=w277:path)
        n128 = call <vilib>:"Open Config Data.vi"("configuration file path"=w277) -> ("error out"=w283:errorcluster, "refnum"=w282:T15)  [unwired: 8 in, 1 out]
        n129 = call-poly <vilib>:"Write Key.vi"("section"="总磷总氮", "error in (no error)"=w283, "value"="VISA Resource", "key"="串口", "refnum"=w282) -> ("error out"=w279:errorcluster, "refnum out"=w275:T15)  [unwired: 4 in, 1 out]
        n130 = call <vilib>:"Close Config Data.vi"("error in (no error)"=w279, "refnum"=w275) -> ()  [unwired: 8 in, 2 out]
      }
      event "启动": Value Change {
        n131 = event-data() -> ()  [unwired: 1 in, 6 out]
        n132 = case shown="默认" "控制命令" {
          tunnel: "控制命令参数" -> [w296 w297]
          tunnel: [w295 w297] -> w284
          frame Default {
            n133 = call "HexToWord.vi"("数组"=w296) -> ("WORD"=w295:u16[])  [unwired: 10 in]
          }
          frame 13 {
          }
        }
        n134 = Swap Bytes(anything="控制命令") -> (byte swapped=w287:u16)
        n135 = call "控制命令区.vi"("控制命令参数"=w284, "控制命令"=w287) -> ("控制命令"=w290:u16[])  [unwired: 9 in]
        n136 = local read "站号"() -> (w289:u16)
        n137 = Bundle("站号"=w289, "控制命令"=w290) -> (w288:cluster{"站号":u16, "控制命令":u16[]})  [unwired: 1 in]
        n138 = Bundle By Name(cluster=cluster{"命令":string, "data":variant} {"命令"="", "data"=variant} ("元素"), "命令"="启动", "data"=w288) -> (w292:cluster{"命令":string, "data":variant})
        n139 = Enqueue Element(queue=w294, element=w292) -> ()  [unwired: 2 in, 3 out]
      }
      event "停止": Value Change {
        n140 = event-data() -> ()  [unwired: 1 in, 6 out]
        n141 = Set Occurrence(w298) -> ()
        n142 = Flush Queue(queue=w301) -> (queue out=w300:refnum<queue>)  [unwired: 1 in, 2 out]
        n143 = Enqueue Element(queue=w300, element=cluster{"命令":string, "data":variant} {"命令"="shutdown", "data"=variant} ("元素")) -> ()  [unwired: 2 in, 3 out]
      }
      event "读测量数据区": Value Change {
        n144 = event-data() -> ()  [unwired: 1 in, 6 out]
        n145 = Bundle By Name(cluster=cluster{"命令":string, "data":variant} {"命令"="", "data"=variant} ("元素"), "命令"="读测量数据区", "data"="站号") -> (w305:cluster{"命令":string, "data":variant})
        n146 = Enqueue Element(queue=w307, element=w305) -> ()  [unwired: 2 in, 3 out]
      }
      event "读状态告警区": Value Change {
        n147 = event-data() -> ()  [unwired: 1 in, 6 out]
        n148 = local read "站号"() -> (w308:u16)
        n149 = Bundle By Name(cluster=cluster{"命令":string, "data":variant} {"命令"="", "data"=variant} ("元素"), "命令"="读状态告警区", "data"=w308) -> (w310:cluster{"命令":string, "data":variant})
        n150 = Enqueue Element(queue=w312, element=w310) -> ()  [unwired: 2 in, 3 out]
      }
      event "读关键参数区": Value Change {
        n151 = event-data() -> ()  [unwired: 1 in, 6 out]
        n152 = local read "站号"() -> (w313:u16)
        n153 = Bundle By Name(cluster=cluster{"命令":string, "data":variant} {"命令"="", "data"=variant} ("元素"), "命令"="读关键参数区", "data"=w313) -> (w315:cluster{"命令":string, "data":variant})
        n154 = Enqueue Element(queue=w317, element=w315) -> ()  [unwired: 2 in, 3 out]
      }
    }
  }
  n155 = while {
    tunnel: w12 -> [w326]
    tunnel: w11 -> [w322]
    stop <- w323 stop-if-true
    n156 = global read "总磷总氮断电保存全局变量.vi" "MB通信方式选择"() -> (w321:enum16{"串口", "TCP"})
    n157 = Wait on Occurrence(2:w326, 3:10000 ("毫秒超时(-1)")) -> (0:w324:bool)  [unwired: 1 in]
    n158 = Not(x=w324) -> (.not. x?=w323:bool)
    n159 = case shown="\"TCP\"" w321 {
      tunnel: [_ w327] -> w318
      frame "串口", Default {
      }
      frame "TCP" {
        n160 = global read "VAR总磷总氮全局变量.vi" "MB session in"() -> (w329:refnum<class "MB_Master.lvclass">)
        n161 = property class="MB_Master"(reference=w329) -> ("Properties:Session Valid"=w328:bool)  [unwired: 1 in, 2 out]
        n162 = Not(x=w328) -> (.not. x?=w327:bool)
      }
    }
    n163 = First Call?() -> (First Call?: T/F=w320:bool)
    n164 = Or(x=w318, y=w320) -> (x .or. y?=w319:bool)
    n165 = case shown="真" w319 {
      tunnel: w322 -> [_ w332]
      frame False {
      }
      frame True {
        n166 = Flush Queue(queue=w332) -> (queue out=w330:refnum<queue>)  [unwired: 1 in, 2 out]
        n167 = Enqueue Element(queue=w330, element=cluster{"命令":string, "data":variant} {"命令"="启用模块", "data"=variant} ("元素")) -> ()  [unwired: 2 in, 3 out]
        n168 = property on="VISA Resource" class="VISAName"("DisabledEnum"=T16."Disabled and Grayed Out" ("禁用")) -> ()  [unwired: 2 in, 2 out]
      }
    }
  }
  n169 = while {
    tunnel: w11 -> [w350]
    tunnel: w14 -> [w349]
    shift-right: [w334] -> _
    shift-left: _ -> [w347]
    tunnel: errorcluster {"status"=FALSE, "code"=0, "source"=""} ("error out") -> [w346]
    tunnel: [w342] -> _
    stop <- w348 stop-if-true
    n170 = Dequeue Element(queue=w350, error in (no error)=w349) -> (queue out=w343:refnum<queue>, element=w344:cluster{"命令":string, "data":variant})  [unwired: 1 in, 2 out]
    n171 = Unbundle By Name(w344) -> ("命令"=w345:string, "data"=w340:variant)
    n172 = case shown="\"读状态告警区\"" w345 {
      tunnel: w340 -> [_ _ _ w377 w388 w405 w423 w472 w492 _]
      tunnel: w343 -> [_ _ _ _ _ _ _ _ _ w505]
      tunnel: [_ _ _ _ _ _ _ _ _ TRUE] -> w348
      tunnel: [w356 w358 w364 w380 w391 w407 w427 w480 w499 w501] -> w334
      tunnel: [w357 w359 w365 w379 w390 w406 w428 w471 w500 w502] -> w342
      tunnel: w347 -> [w356 _ w364 w376 w387 w404 w422 w475 w495 w501]
      tunnel: w346 -> [w357 _ w366 w373 w384 w401 w420 w476 w496 w503]
      tunnel: [_ _ _ w368 w381 w395 w410 w465 w486 _] -> w335
      frame Default {
      }
      frame "启用模块" {
        n173 = call "总磷总氮MB_api.vi"("STEP"=enum16{"open", "read", "write", "close"}."open") -> ("error out"=w359:errorcluster, "MB session out"=w358:refnum<class "MB_Master.lvclass">)  [unwired: 8 in, 1 out]
      }
      frame "停用模块" {
        n174 = call-dynamic "Close Session.vi"("error in (no error)"=w366, "MB session in"=w364) -> ("error out"=w363:errorcluster)  [unwired: 9 in]
        n175 = call "总磷总氮MB_api.vi"("STEP"=enum16{"open", "read", "write", "close"}."close", "Error in"=w363) -> ("error out"=w362:errorcluster)  [unwired: 7 in, 2 out]
        n176 = call <vilib>:"Clear Errors.vi"("error in (no error)"=w362) -> ("error out"=w365:errorcluster)  [unwired: 5 in, 1 out]
      }
      frame "启动" {
        n177 = Variant To Data(type=cluster{"站号":u16, "控制命令":u16[]} {"站号"=0, "控制命令"=[]} ("输出簇"), Variant=w377) -> (data=w371:cluster{"站号":u16, "控制命令":u16[]})  [unwired: 1 in, 1 out]
        n178 = Unbundle By Name(w371) -> ("站号"=w368:u16, "控制命令"=w369:u16[])
        n179 = property class="MB_Master"(reference=w376, error in=w373, "Properties:Slave ID"=w368) -> (reference out=w375:refnum<class "MB_Master.lvclass">, error out=w374:errorcluster)
        n180 = Index Array(array=w369) -> (element=w370:u16)  [unwired: 1 in]
        n181 = Swap Bytes(anything=w370) -> (byte swapped=w367:u16)
        n182 = global write "VAR总磷总氮全局变量.vi" "控制命令"(w367) -> ()
        n183 = call <vilib>:"Write Multiple Registers.vi"("error in (no error)"=w374, "values"=w369, "starting address"=u16 4608, "MB session in"=w375) -> ("error out"=w379:errorcluster, "MB session out"=w380:refnum<class "MB_Master.lvclass">)  [unwired: 6 in]
      }
      frame "盲样测试" {
        n184 = Variant To Data(type=u8 0, Variant=w388) -> (data=w381:u8)  [unwired: 1 in, 1 out]
        n185 = property class="MB_Master"(reference=w387, error in=w384, "Properties:Slave ID"=w381) -> (reference out=w386:refnum<class "MB_Master.lvclass">, error out=w385:errorcluster)
        n186 = case shown="默认" w381 {
          tunnel: [u16[] [] ("values") u16[] [33539, 0] ("values") u16[] [23555, 0] ("values")] -> w383
          frame Default {
          }
          frame 1 {
            # "总磷盲样测试命令"
          }
          frame 3 {
            # "氨氮盲样测试"
          }
        }
        n187 = call <vilib>:"Write Multiple Registers.vi"("error in (no error)"=w385, "values"=w383, "starting address"=u16 24592, "MB session in"=w386) -> ("error out"=w390:errorcluster, "MB session out"=w391:refnum<class "MB_Master.lvclass">)  [unwired: 6 in]
      }
      frame "debug" {
        n188 = Variant To Data(type=cluster{"站号":u16, "控制命令":u16[]} {"站号"=0, "控制命令"=[]} ("输出簇"), Variant=w405) -> (data=w399:cluster{"站号":u16, "控制命令":u16[]})  [unwired: 1 in, 1 out]
        n189 = Unbundle By Name(w399) -> ("站号"=w395:u16, "控制命令"=w397:u16[])
        n190 = property class="MB_Master"(reference=w404, error in=w401, "Properties:Slave ID"=w395) -> (reference out=w403:refnum<class "MB_Master.lvclass">, error out=w402:errorcluster)
        n191 = Index Array(array=w397) -> (element=w398:u16)  [unwired: 1 in]
        n192 = global write "VAR总磷总氮全局变量.vi" "控制命令"(w398) -> ()
        n193 = call <vilib>:"Write Multiple Registers.vi"("error in (no error)"=w402, "values"=w397, "starting address"=u16 24594, "MB session in"=w403) -> ("error out"=w406:errorcluster, "MB session out"=w407:refnum<class "MB_Master.lvclass">)  [unwired: 6 in]
      }
      frame "读测量数据区" {
        n194 = Variant To Data(type=u8 1 ("Slave ID"), Variant=w423) -> (data=w410:u8)  [unwired: 1 in, 1 out]
        n195 = property class="MB_Master"(reference=w422, error in=w420, "Properties:Slave ID"=w410) -> (reference out=w421:refnum<class "MB_Master.lvclass">, error out=w419:errorcluster)
        n196 = global read "VAR总磷总氮全局变量.vi" "测量数据区数组"() -> (w416:T6)
        n197 = call <vilib>:"Read Holding Registers.vi"("error in (no error)"=w419, "quantity"=u16 107, "starting address"=u16 4096, "MB session in"=w421) -> ("error out"=w428:errorcluster, "Registers"=w418:u16[], "MB session out"=w427:refnum<class "MB_Master.lvclass">)  [unwired: 5 in]
        n198 = call "id参数转换.vi"("id"=w410) -> ("数组资源索引"=w409:i32)  [unwired: 9 in, 1 out]
        n199 = call "测量数据区.vi"("数组"=w418) -> ("测量数据区"=w415:T5)  [unwired: 10 in]
        "测量数据区" <- w415
        n200 = Index Array(array=w416, index #1=w409, index #2=1 ("索引")) -> (element #1=w417:T5, element #2=w411:T5, element #3=w408:T5)  [unwired: 1 in]
        n201 = global write "VAR总磷总氮全局变量.vi" "测量数据区"(w415) -> ()
        n202 = case shown="0, 默认" w410 {
          tunnel: w415 -> [w429 w434 w458 w460 w462]
          tunnel: w418 -> [_ w442 w459 w461 w463]
          tunnel: w417 -> [_ w435 _ _ _]
          tunnel: [w429 w437 w458 w460 w462] -> w414
          tunnel: w411 -> [_ w432 _ _ _]
          tunnel: w408 -> [_ w431 _ _ _]
          frame 0, Default {
          }
          frame 1 {
            n203 = global read "VAR总磷总氮全局变量.vi" "模块名称"() -> (w441:string)
            n204 = Search and Replace String(input string=w441, search string="总磷" ("搜索字符串")) -> (result string=w438:string, offset past replacement=w439:i32)  [unwired: 6 in, 2 out]
            n205 = case shown="默认" w439 {
              tunnel: w438 -> [_ w448]
              tunnel: [_ w445] -> w436
              tunnel: [_ w443] -> w433
              frame -1 {
              }
              frame Default {
                n206 = Search and Replace String(input string=w448, search string="总氮" ("搜索字符串")) -> (offset past replacement=w451:i32)  [unwired: 6 in, 3 out]
                n207 = Search and Replace String(input string=w448, search string="氨氮" ("搜索字符串")) -> (offset past replacement=w446:i32)  [unwired: 6 in, 3 out]
                n208 = Not Equal?(x=w451, y=-1) -> (x != y?=w443:bool)
                n209 = Not Equal?(x=w446, y=-1) -> (x != y?=w444:bool)
                n210 = Or(x=w444, y=w443) -> (x .or. y?=w445:bool)
              }
            }
            n211 = Select(t=w432, s=w433, f=w431) -> (s? t:f=w430:T5)
            n212 = case shown="真" w436 {
              tunnel: [w453 w457] -> w437
              tunnel: w435 -> [_ w456]
              tunnel: w430 -> [_ w455]
              tunnel: w434 -> [w453 w454]
              frame False {
              }
              frame True {
                # "启动总磷总氮时间自动对齐"
                n213 = call "数据时间对齐.vi"("待对齐时间"=w454, "对齐参考时间"=w455, "已对齐时间输入"=w456) -> ("已对齐时间输出"=w457:T5)  [unwired: 8 in]
              }
            }
            "总磷测量数据区" <- w442
          }
          frame 2 {
            "总氮测量数据区" <- w459
          }
          frame 3 {
            "氨氮测量数据区" <- w461
          }
          frame 22 {
            "COD测量数据区" <- w463
          }
        }
        n214 = Replace Array Subset(array=w416, new element=w414, index=w409) -> (w413:T6)
        n215 = global write "VAR总磷总氮全局变量.vi" "测量数据区数组"(w413) -> ()
      }
      frame "读状态告警区" {
        n216 = Variant To Data(type=u8 1 ("Slave ID"), Variant=w472) -> (data=w465:u8)  [unwired: 1 in, 1 out]
        n217 = property class="MB_Master"(reference=w475, error in=w476, "Properties:Slave ID"=w465) -> (reference out=w474:refnum<class "MB_Master.lvclass">, error out=w473:errorcluster)
        n218 = call "id参数转换.vi"("id"=w465) -> ("数组资源索引"=w464:i32)  [unwired: 9 in, 1 out]
        n219 = call <vilib>:"Read Holding Registers.vi"("error in (no error)"=w473, "quantity"=u16 29, "starting address"=u16 4224, "MB session in"=w474) -> ("error out"=w471:errorcluster, "Registers"=w469:u16[], "MB session out"=w480:refnum<class "MB_Master.lvclass">)  [unwired: 5 in]
        n220 = global read "VAR总磷总氮全局变量.vi" "状态告警区数组"() -> (w468:T8)
        n221 = call "状态告警区.vi"("数组"=w469) -> ("状态告警区"=w467:T4)  [unwired: 10 in]
        "状态告警区" <- w467
        n222 = global write "VAR总磷总氮全局变量.vi" "状态告警区"(w467) -> ()
        n223 = Unbundle By Name(w467) -> ("id"=w470:u16)
        n224 = Replace Array Subset(array=w468, new element=w467, index=w464) -> (w466:T8)
        n225 = case shown="3" w470 {
          tunnel: w467 -> [_ _ _ _ _]
          tunnel: w469 -> [_ w481 w482 w483 w484]
          frame 0, Default {
          }
          frame 1, 131 {
            "总磷状态告警区" <- w481
          }
          frame 2, 76 {
            "总氮状态告警区" <- w482
          }
          frame 3 {
            "氨氮状态告警区" <- w483
          }
          frame 22 {
            "COD状态告警区" <- w484
          }
        }
        n226 = global write "VAR总磷总氮全局变量.vi" "状态告警区数组"(w466) -> ()
      }
      frame "读关键参数区" {
        n227 = Variant To Data(type=u8 1 ("Slave ID"), Variant=w492) -> (data=w486:u8)  [unwired: 1 in, 1 out]
        n228 = property class="MB_Master"(reference=w495, error in=w496, "Properties:Slave ID"=w486) -> (reference out=w494:refnum<class "MB_Master.lvclass">, error out=w493:errorcluster)
        n229 = call "id参数转换.vi"("id"=w486) -> ("数组资源索引"=w485:i32)  [unwired: 9 in, 1 out]
        n230 = call <vilib>:"Read Holding Registers.vi"("error in (no error)"=w493, "quantity"=u16 19, "starting address"=u16 4256, "MB session in"=w494) -> ("error out"=w500:errorcluster, "Registers"=w490:u16[], "MB session out"=w499:refnum<class "MB_Master.lvclass">)  [unwired: 5 in]
        n231 = global read "VAR总磷总氮全局变量.vi" "关键参数区数组"() -> (w489:T7)
        n232 = call "关键参数区.vi"("数组"=w490) -> ("关键参数区"=w488:T3)  [unwired: 10 in]
        "关键参数区" <- w488
        n233 = global write "VAR总磷总氮全局变量.vi" "关键参数区"(w488) -> ()
        n234 = Replace Array Subset(array=w489, new element=w488, index=w485) -> (w487:T7)
        n235 = global write "VAR总磷总氮全局变量.vi" "关键参数区数组"(w487) -> ()
      }
      frame "shutdown" {
        n236 = call-dynamic "Close Session.vi"("error in (no error)"=w503, "MB session in"=w501) -> ("error out"=w502:errorcluster)  [unwired: 9 in]
        n237 = Flush Queue(queue=w505) -> (queue out=w504:refnum<queue>)  [unwired: 1 in, 2 out]
        n238 = Release Queue(queue=w504) -> ()  [unwired: 2 in, 3 out]
      }
    }
    n239 = global write "VAR总磷总氮全局变量.vi" "MB session in"(w334) -> ()
    n240 = Unbundle By Name(w342) -> ("status"=w338:bool)
    n241 = Not(x=w338) -> (.not. x?=w341:bool)
    "status" <- w341
    n242 = call <vilib>:"Boolean Crossing PtByPt.vi"("direction"=enum16{"either", "false-true", "true-false"}."false-true", "input"=w338) -> ("crossing"=w337:bool)  [unwired: 1 in]
    n243 = call "id参数转换.vi"("id"=w335) -> ("table输出"=w339:string)  [unwired: 9 in, 1 out]
    n244 = case shown="真" w337 {
      tunnel: w339 -> [_ w354]
      frame False {
      }
      frame True {
        n245 = Get Date/Time In Seconds() -> (seconds since 1Jan1904=w353:timestamp)
        n246 = Bundle By Name(cluster=T17 {"时间标识"=timestamp(0 s since 1904-01-01), "设备"="", "日志信息"="", "备注"=""} ("data in"), "时间标识"=w353, "设备"=w354, "日志信息"="通讯告警") -> (w352:T17)
        n247 = call "总磷总氮报警信息.vi"("data in"=w352) -> ()  [unwired: 10 in, 1 out]
      }
    }
    n248 = global write "VAR总磷总氮全局变量.vi" "通讯状态"(w341) -> ()
  }
